vi "AutonSelectionStore.vi"(10 "Update?":bool, 11 "AutonSelectionIn":string) -> (3 "AutonSelectionOut":string)   [LabVIEW 2017]
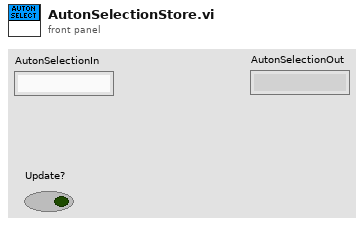
[diagram p1: front panel]
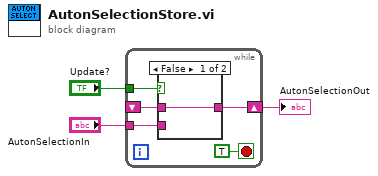
[diagram p0: block diagram]
diagram:
  n1 = while {
    tunnel: "Update?" -> [w7]
    tunnel: "AutonSelectionIn" -> [w6]
    shift-right: [w5] -> w1
    shift-left: _ -> [w4]
    stop <- TRUE stop-if-true
    n2 = case shown="False" w7 {
      tunnel: w6 -> [_ w10]
      tunnel: [w9 w10] -> w5
      tunnel: w4 -> [w9 _]
      frame False {
      }
      frame True {
      }
    }
  }
  "AutonSelectionOut" <- w1
